vi "Delete TTL.vi"(0 "Tosca in":refnum<class "Parameters.lvclass">, 7 "Name":string, 11 "error in (no error)":errorcluster) -> (4 "Tosca out":refnum<class "Parameters.lvclass">, 15 "error out":errorcluster)   [LabVIEW 2015, in "Parameters.lvclass"]
uses:
  Parameters.lvclass
  Parameters.lvclass/Parameters.ctl
  State/State.lvclass
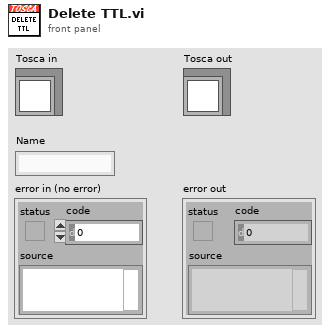
[diagram p1: front panel]
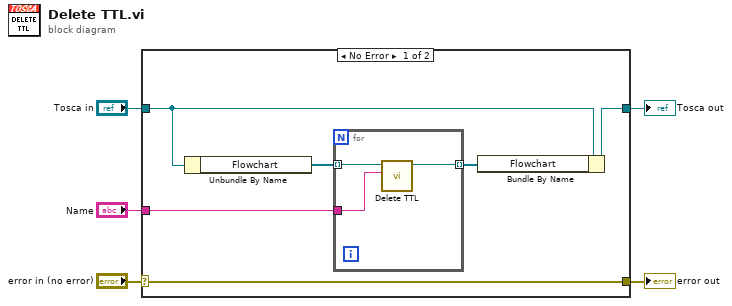
[diagram p0: block diagram]
diagram:
  n1 = case shown="No Error" "error in (no error)" {
    selector: "error in (no error)" -> [w11 w16]
    tunnel: [w11 w16] -> w4
    tunnel: [w8 w15] -> w2
    tunnel: "Tosca in" -> [w10 w15]
    tunnel: "Name" -> [w7 _]
    frame No Error {
      n2 = Unbundle By Name(w10) -> ("Flowchart"=w9:refnum<class "State.lvclass">[])
      n3 = for {
        tunnel: w9 -> [w14] mode=indexing
        tunnel: w7 -> [w13]
        tunnel: [w12] -> w6 mode=indexing
        n4 = call "Delete TTL.vi"("Name"=w13, "State in"=w14) -> ("State out"=w12:refnum<class "State.lvclass">)  [unwired: 8 in, 1 out]
      }
      n5 = Bundle By Name(cluster=w10, "Flowchart"=w6) -> (w8:refnum<class "Parameters.lvclass">)
    }
    frame Error {
    }
  }
  "error out" <- w4
  "Tosca out" <- w2
